vi "mqttCmdBuildVarHdr.vi"(0 "_mqtt in":refnum<class "mqttCmdPublish.lvclass">, 11 "error in (no error)":errorcluster) -> (4 "_mqtt out":refnum<class "mqttCmdPublish.lvclass">, 8 "variableHeader":u8[](array[numeric]) format="%02x", 15 "error out":errorcluster)   [LabVIEW 2019, in "mqttCmdPublish.lvclass"]
uses:
  mqttCmdPublish.lvclass
  D:/Wade/Project/IoT_Project/MQTT_Project/mqtt_lv2013/mqtt Folder/src/class/mqtt/mqttCmd/mqttCmd.lvclass
  mqttCmd.lvclass/mqttCmd.ctl
  mqttCmdPublish.lvclass/mqttCmdPublish.ctl
  mqttCmd.lvclass
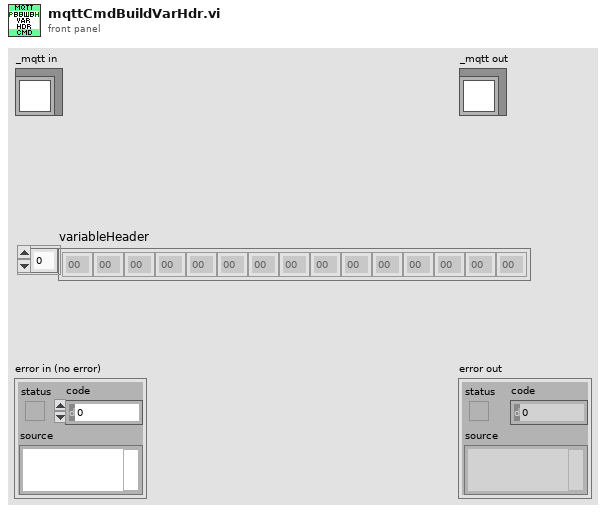
[diagram p1: front panel]
types:
  T1 = typedef "mqttQOSlevel.ctl" = enum8{"At most once", "At least once", "Exactly once", "Reserved"}
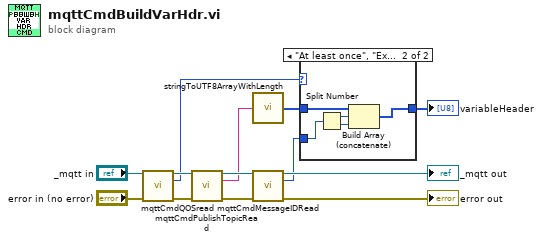
[diagram p0: block diagram]
diagram:
  n1 = call "mqttCmdQOSread.vi"("mqttBrokerCommand in"="_mqtt in", "error in (no error)"="error in (no error)") -> ("mqttBrokerCommand out"=w3:refnum<class "mqttCmdPublish.lvclass">, "QoS"=w1:T1, "error out"=w2:errorcluster)  [unwired: 11 in]
  n2 = call "mqttCmdPublishTopicRead.vi"("mqttPublish in"=w3, "error in (no error)"=w2) -> ("mqttPublish out"=w8:refnum<class "mqttCmdPublish.lvclass">, "topic"=w6:string, "error out"=w7:errorcluster)  [unwired: 11 in]
  n3 = call "stringToUTF8ArrayWithLength.vi"("string"=w6) -> ("UTF8[]"=w9:u8[])  [unwired: 14 in]
  n4 = call "mqttCmdMessageIDRead.vi"("mqttBrokerCommand in"=w8, "error in (no error)"=w7) -> ("mqttBrokerCommand out"=→"_mqtt out":refnum<class "mqttCmdPublish.lvclass">, "messageID"=w11:u16, "error out"=→"error out":errorcluster)  [unwired: 11 in]
  n5 = case shown="\"At least once\", \"Exactly once\"" w1 {
    tunnel: w11 -> [_ w17]
    tunnel: [w14 w16] -> w10
    tunnel: w9 -> [w14 w15]
    frame "At most once", Default {
    }
    frame "At least once", "Exactly once" {
      n6 = Split Number(x=w17) -> (hi(x)=w18:u8, lo(x)=w19:u8)
      n7 = Build Array (concatenate)(w15, w18, w19) -> (w16:u8[])
    }
  }
  "variableHeader" <- w10
